vi "chrmawsd.vi"() -> ()   [LabVIEW 2011]
uses:
  <vilib>/Utility/file.llb/Write To Spreadsheet File (string).vi
  <vilib>/Utility/file.llb/Read From Spreadsheet File (DBL).vi
  <vilib>/ptbypt/NI_PtbyPt.lvlib
panel:
  out "sum 2":dbl
  out "sum":dbl
  out "x*y":dbl[](array[numeric])
  out "mean 2":dbl
  out "x-y":dbl[](array[numeric])
  out "mean":dbl format="%0.2f"
  out "first row":dbl[](array[numeric]) format="%0.3f"
  in  "Name of File":string
  out "error out":errorcluster
  in  "resource name 2":refnum<visa-resource-name> caption="resource name"
  in  "Type (V_RMS)":i32(ring) items=["V_THD"=3, "V_PEAK-"=2, "V_PEAK+"=1, "V_RMS"=0]
  in  "Type (I_RMS)":i32(ring) items=["I_THD"=5, "I_CRESTFACTOR"=4, "I_INRUSH"=3, "I_PEAK-"=2, "I_PEAK+"=1, "I_RMS"=0]
  in  "Type (P_REAL)":i32(ring) items=["P_ENERGY"=4, "P_FACTOR"=3, "P_REACTIVE"=2, "P_APPARENT"=1, "P_REAL"=0]
  out "Current Data Point":i32
  in  "Press to Stop":bool
  out "appended array":string[](array[string])
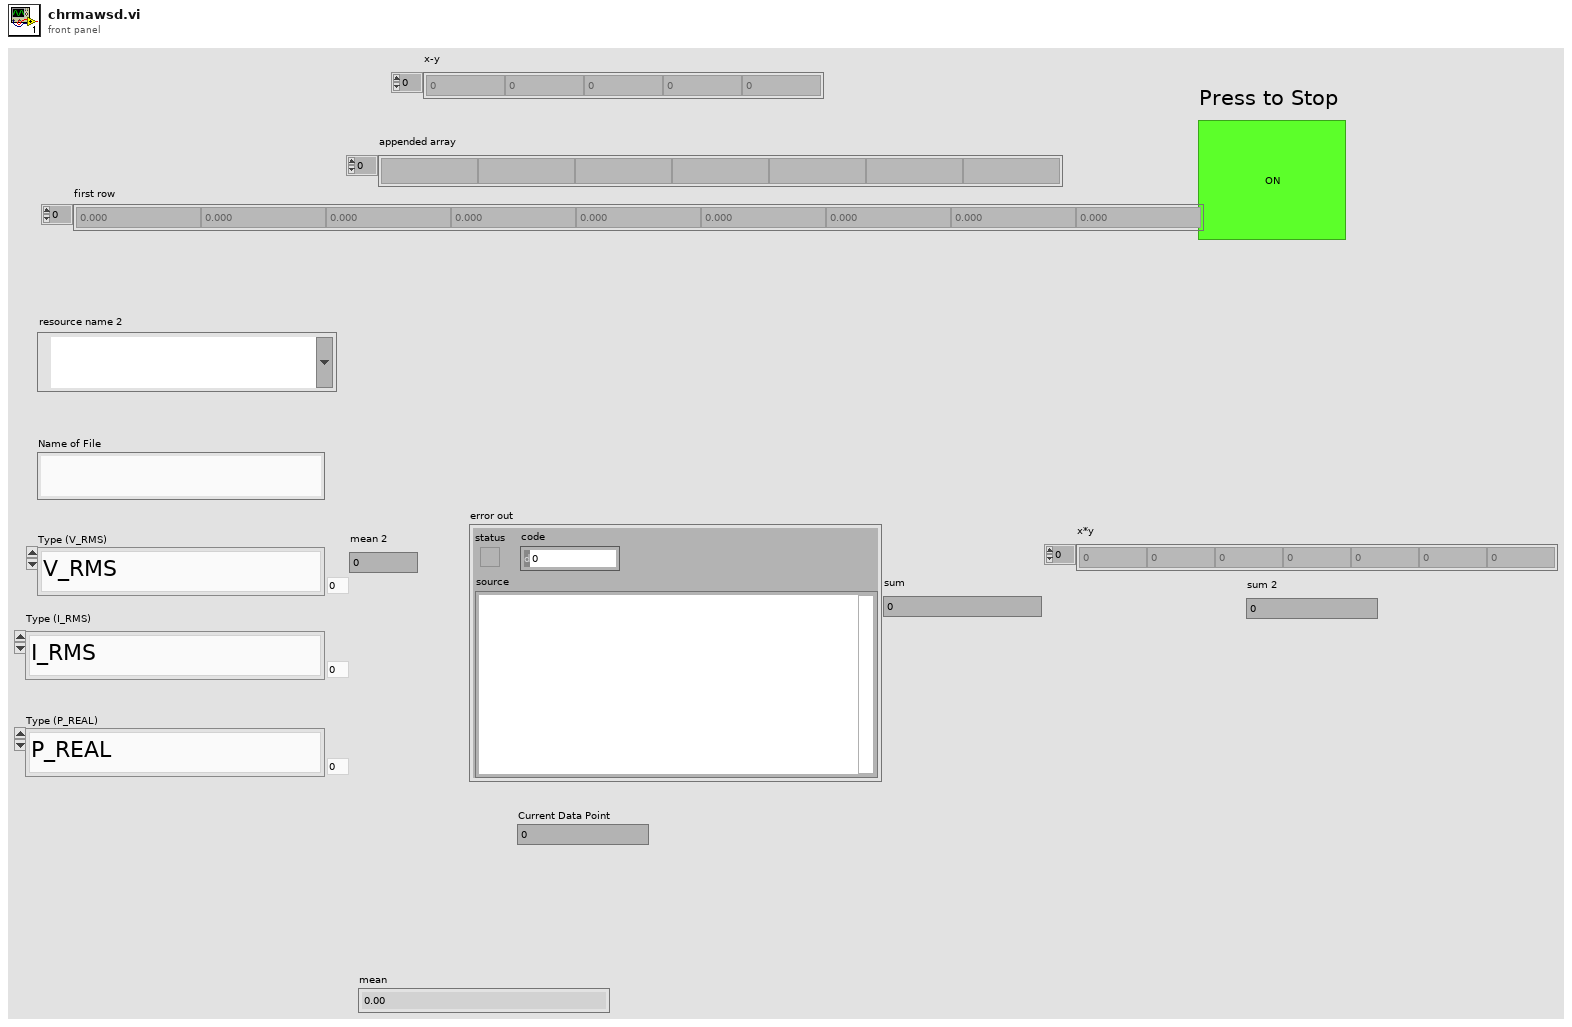
[diagram p1: front panel]
types:
  T1 = enum16{"open", "replace", "create", "open or create", "replace or create", "replace or create with confirmation"}
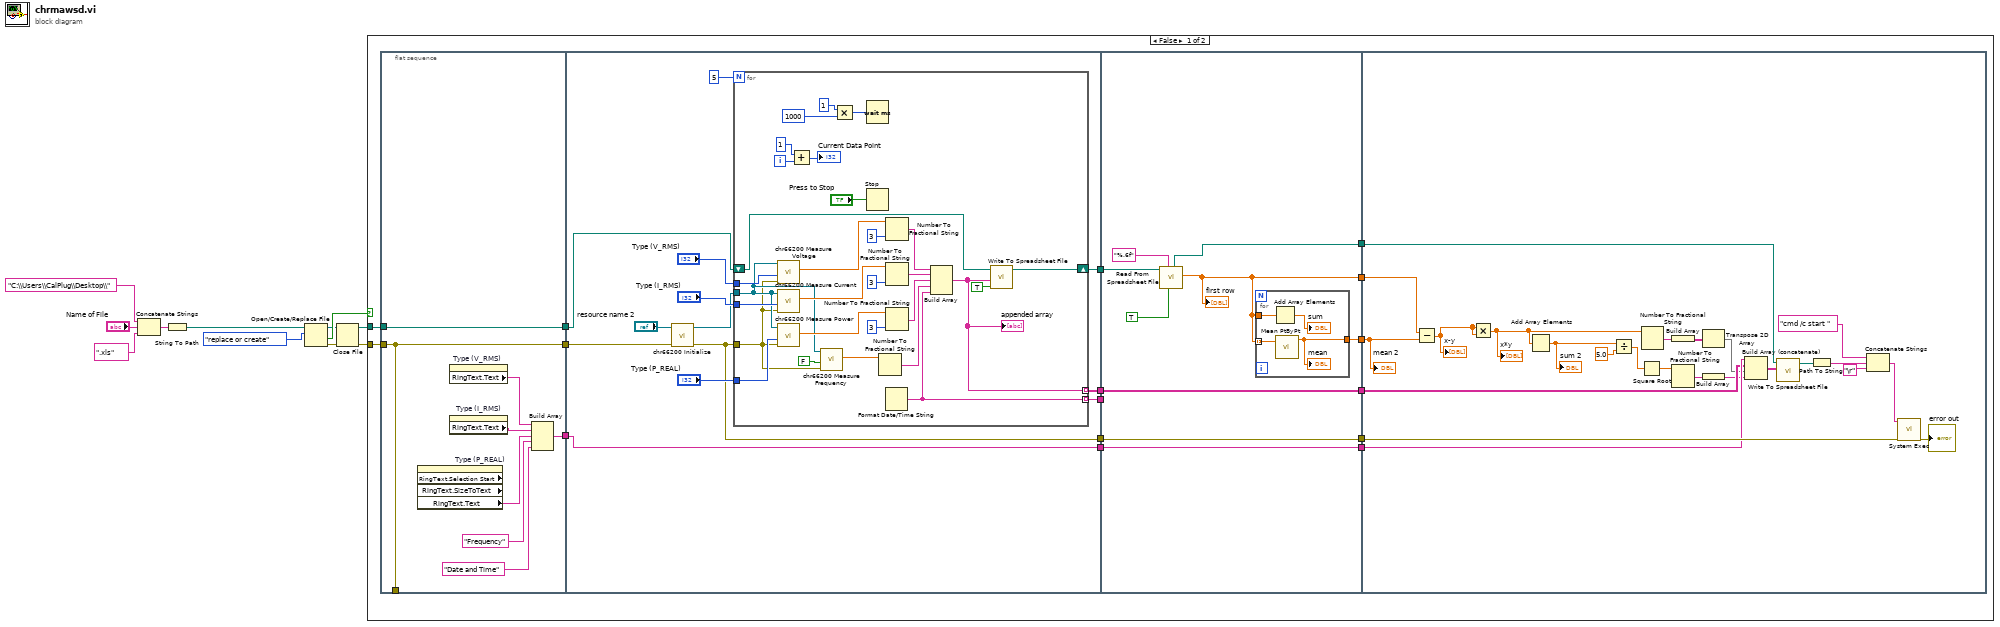
[diagram p0: block diagram]
diagram:
  n1 = Concatenate Strings("C:\\Users\\CalPlug\\Desktop\\" ("string"), "Name of File", ".xls" ("string")) -> (w11:string)
  n2 = String To Path(string=w11) -> (path=w10:path)
  n3 = Open/Create/Replace File(file path (use dialog)=w10, operation (0:open)=T1."replace or create") -> (refnum out=w4:refnum<file>, cancelled=w5:bool, error out=w3:errorcluster)  [unwired: 4 in]
  n4 = Close File(refnum=w4, error in=w3) -> (path=w1:path, error out=w2:errorcluster)
  n5 = case shown="False" w5 {
    tunnel: w2 -> [w24 _]
    tunnel: w1 -> [w22 _]
    frame False {
      n6 = flat-sequence {
        tunnel: [w32] -> w27
        tunnel: [w32] -> _
        tunnel: w24 -> [w32]
        tunnel: [w30] -> w23
        tunnel: w22 -> [w30]
        tunnel: [w29] -> w21
        tunnel: w27 -> [w43]
        tunnel: [w42] -> w26
        tunnel: [w41] -> w25
        tunnel: w23 -> [w39]
        tunnel: w21 -> [w38]
        tunnel: [w38] -> w16
        tunnel: [w37] -> w14
        tunnel: [w36] -> w13
        tunnel: w26 -> [w85]
        tunnel: w25 -> [w84]
        tunnel: [w84] -> w20
        tunnel: [w83] -> w19
        tunnel: [w79] -> w18
        tunnel: [w82] -> w17
        tunnel: w16 -> [w81]
        tunnel: [w81] -> w15
        tunnel: w14 -> [_]
        tunnel: w13 -> [w80]
        tunnel: [w80] -> w12
        tunnel: w20 -> [w109]
        tunnel: w19 -> [w108]
        tunnel: w18 -> [w106]
        tunnel: w17 -> [w105]
        tunnel: w15 -> [w101]
        tunnel: w12 -> [w100]
        frame #0 {
          n7 = property on="Type (P_REAL)" class="Ring (strict)" props=["RingText", "Selection Start", "RingText", "SizeToText", "RingText", "Text"]() -> ("RingText.Text"=w35:string)  [unwired: 2 in, 4 out]
          n8 = property on="Type (V_RMS)" class="Ring (strict)"() -> ("RingText.Text"=w28:string)  [unwired: 2 in, 2 out]
          n9 = property on="Type (I_RMS)" class="Ring (strict)"() -> ("RingText.Text"=w34:string)  [unwired: 2 in, 2 out]
          n10 = Build Array(w28, w34, w35, "Frequency" ("element"), "Date and Time" ("element")) -> (w29:string[])
        }
        frame #1 {
          n11 = call <instrlib>:"chr66200 Initialize.vi"("error in (no error)"=w43, "resource name"="resource name 2") -> ("error out"=w41:errorcluster, "instrument handle out"=w45:refnum<visa-resource-name>)  [unwired: 8 in]
          n12 = for {
            N: u32 5 ("seconds to wait") -> [_]
            tunnel: w45 -> [w59]
            tunnel: w41 -> [w54]
            tunnel: "Type (I_RMS)" -> [w77]
            tunnel: "Type (V_RMS)" -> [w76]
            tunnel: "Type (P_REAL)" -> [w75]
            shift-right: [w74] -> w42
            shift-left: w39 -> [w51]
            tunnel: [w50] -> w37 mode=indexing
            tunnel: [w49] -> w36 mode=indexing
            i -> [w66]
            n13 = call <instrlib>:"chr66200 Measure Voltage.vi"("error in (no error)"=w54, "Type (V_RMS)"=w76, "instrument handle"=w59) -> ("Read Value"=w72:dbl)  [unwired: 6 in, 2 out]
            n14 = call <instrlib>:"chr66200 Measure Current.vi"("error in (no error)"=w54, "Type (I_RMS)"=w77, "instrument handle"=w59) -> ("Read Value"=w71:dbl)  [unwired: 6 in, 2 out]
            n15 = call <instrlib>:"chr66200 Measure Power.vi"("error in (no error)"=w54, "Type (P_REAL)"=w75, "instrument handle"=w59) -> ("Read Value"=w70:dbl)  [unwired: 6 in, 2 out]
            n16 = Add(x=1, y=w66) -> (x+y=→"Current Data Point":i32)
            n17 = call <instrlib>:"chr66200 Measure Frequency.vi"("error in (no error)"=w54, "Measure Fetch (Fetch)"=FALSE, "instrument handle"=w59) -> ("Read Value"=w57:dbl)  [unwired: 6 in, 2 out]
            n18 = Multiply(x=u32 1 ("Interval of Data Collection (sec)"), y=u32 1000) -> (x*y=w62:u32)
            n19 = Wait (ms)(milliseconds to wait=w62) -> ()  [unwired: 1 out]
            n20 = Stop(stop? (T)="Press to Stop") -> ()
            n21 = Number To Fractional String(number=w57) -> (F-format string=w55:string)  [unwired: 3 in]
            n22 = Format Date/Time String() -> (date/time string=w50:string)  [unwired: 3 in]
            n23 = Number To Fractional String(number=w72, precision (6)=i16 3) -> (F-format string=w61:string)  [unwired: 2 in]
            n24 = Number To Fractional String(number=w71, precision (6)=i16 3) -> (F-format string=w60:string)  [unwired: 2 in]
            n25 = Number To Fractional String(number=w70, precision (6)=i16 3) -> (F-format string=w56:string)  [unwired: 2 in]
            n26 = Build Array(w61, w60, w56, w55, w50) -> (w49:string[])
            "appended array" <- w49
            n27 = call-poly <vilib>:"Write To Spreadsheet File.vi"("append to file? (new file:F)"=TRUE, "1D data"=w49, "file path (dialog if empty)"=w51) -> ("new file path (Not A Path if cancelled)"=w74:path)  [unwired: 5 in]
          }
        }
        frame #2 {
          n28 = call-poly <vilib>:"Read From Spreadsheet File.vi"("transpose (no:F)"=TRUE, "format (%.3f)"="%.6f", "file path (dialog if empty)"=w85) -> ("first row"=w79:dbl[], "new file path (Not A Path if cancelled)"=w83:path)  [unwired: 4 in, 3 out]
          "first row" <- w79
          n29 = for {
            tunnel: w79 -> [w89]
            tunnel: [w90] -> w82
            tunnel: w79 -> [w88] mode=indexing
            n30 = Add Array Elements(numeric array=w89) -> (sum=→"sum":dbl)
            n31 = call <vilib>:"Mean PtByPt.vi"("x"=w88) -> ("mean"=w90:dbl)  [unwired: 3 in, 1 out]
            "mean" <- w90
          }
        }
        frame #3 {
          n32 = Subtract(x=w106, y=w105) -> (x-y=w98:dbl[])
          "x-y" <- w98
          n33 = Multiply(x=w98, y=w98) -> (x*y=w97:dbl[])
          "x*y" <- w97
          n34 = Add Array Elements(numeric array=w97) -> (sum=w96:dbl)
          "sum 2" <- w96
          n35 = Divide(x=w96, y=5.0) -> (x/y=w94:dbl)
          n36 = Square Root(x=w94) -> (sqrt(x)=w93:dbl)
          n37 = Number To Fractional String(number=w97) -> (F-format string=w102:string[])  [unwired: 3 in]
          n38 = Build Array(w102) -> (w103:string[][])
          n39 = Number To Fractional String(number=w93) -> (F-format string=w92:string)  [unwired: 3 in]
          n40 = Transpose 2D Array(2D array=w103) -> (transposed array=w99:string[][])
          n41 = Build Array(w92) -> (w91:string[])
          n42 = Build Array (concatenate)(w101, w100, w99, w91) -> (w104:string[][])
          n43 = call-poly <vilib>:"Write To Spreadsheet File.vi"("2D data"=w104, "file path (dialog if empty)"=w108) -> ("new file path (Not A Path if cancelled)"=w107:path)  [unwired: 6 in]
          n44 = Path To String(path=w107) -> (string=w111:string)
          n45 = Concatenate Strings("cmd /c start " ("string"), w111, "\r") -> (w113:string)
          n46 = call <vilib>:"System Exec.vi"("error in (no error)"=w109, "command line"=w113) -> ("error out"=→"error out":errorcluster)  [unwired: 6 in, 3 out]
          "mean 2" <- w105
        }
      }
    }
    frame True {
    }
  }
